vi "Read connection ID.vi"(8 "error in (no error)":errorcluster, 11 "TCPIP in":refnum<class "TCPIP.lvclass">) -> (0 "error out":errorcluster, 2 "connection ID":refnum<k5>, 3 "TCPIP out":refnum<class "TCPIP.lvclass">)   [LabVIEW 2018, in "TCPIP.lvclass"]
uses:
  TCPIP.lvclass
  TCPIP.lvclass/TCPIP.ctl
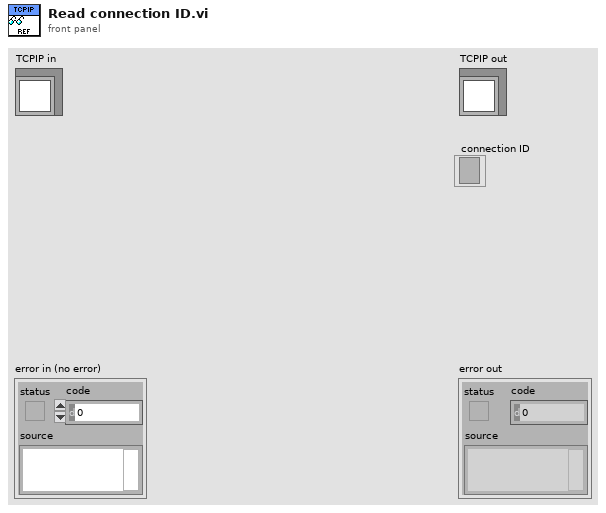
[diagram p1: front panel]
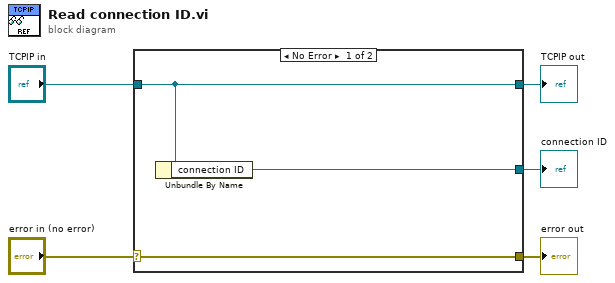
[diagram p0: block diagram]
diagram:
  n1 = case shown="No Error" "error in (no error)" {
    selector: "error in (no error)" -> [w8 w9]
    tunnel: [w8 w9] -> w4
    tunnel: [w7 w10] -> w2
    tunnel: "TCPIP in" -> [w7 w10]
    tunnel: [w6 _] -> w1
    frame No Error {
      n2 = Unbundle By Name(w7) -> ("connection ID"=w6:refnum<k5>)
    }
    frame Error {
    }
  }
  "error out" <- w4
  "TCPIP out" <- w2
  "connection ID" <- w1
